vi "Blockchain test.vi"() -> ()   [LabVIEW 2013]
uses:
  JSONtext.lvlib
  <vilib>/gmath/NI_Gmath.lvlib
  <vilib>/addons/JSON API/Get Polymorphic/JSON GetSet.lvlib
  <vilib>/addons/JSON API/JSON Value/Set from JSON string.vi
  <vilib>/addons/JSON API/JSON Value/JSON Value.lvclass
  <vilib>/addons/JSON API/Variant JSON/Get as Variant.vi
  <vilib>/addons/JSON API/Variant JSON/Variant JSON.lvlib
panel:
  out "x = y? 2":T1
  out "Cluster 2":T2={"A 6"=34, "T 1"="L", "A"=3, "T 3"="", "T 4"="", "A 2"=1.23456, "T 5"="Test \"quote\",\nand newline.", "T 6"="sdfsdf", "A 3"=34, "Cluster 2"={"T 1"="SubCluster", "T 2"="Test \"quote\",\nand newline.", "A"=34, "T 3"="Test \"quote\",\nand newline.", "T 4"="Test \"quote\",\nand newline.", "A 2"=34, "T 5"="Test \"quote\",\nand newline.", "T 6"="Test \"quote\",\nand newline.", "A 3"=34}, "Array"=[1.23456, 1.23456, 1.23456, 1.23456, 1.23456, 1.23456, 1.23456, 1.23456, 1.23456, 1.23456, 1.23456, 1.23456, 2.23456]}
  in  "Other JSON Library":bool
  out "mean":dbl format="%.3p"
  out "length":i32
  out "Variant out":variant
  out "To Variant":dbl[](array[numeric]) format="%#_3p"
  in  "Cluster":T2={"A 6"=34, "T 1"="Line 1", "A"=34, "T 3"="{\"T\":123}", "T 4"="sdfsdfdsfsdf", "A 2"=1.23456, "T 5"="Test \"quote\",\nand newline.", "T 6"="sdfsdf", "A 3"=34, "Cluster 2"={"T 1"="SubCluster", "T 2"="Test \"quote\",\nand newline.", "A"=34, "T 3"="Test \"quote\",\nand newline.", "T 4"="Test \"quote\",\nand newline.", "A 2"=34, "T 5"="Test \"quote\",\nand newline.", "T 6"="Test \"quote\",\nand newline.", "A 3"=34}, "Array"=[1.23, 1.23, 1.23, 1.23, 1.23, 1.23, 1.23, 1.23, 1.23, 1.23, 2.23]}
  out "<JSON>":string
  out "error out":errorcluster
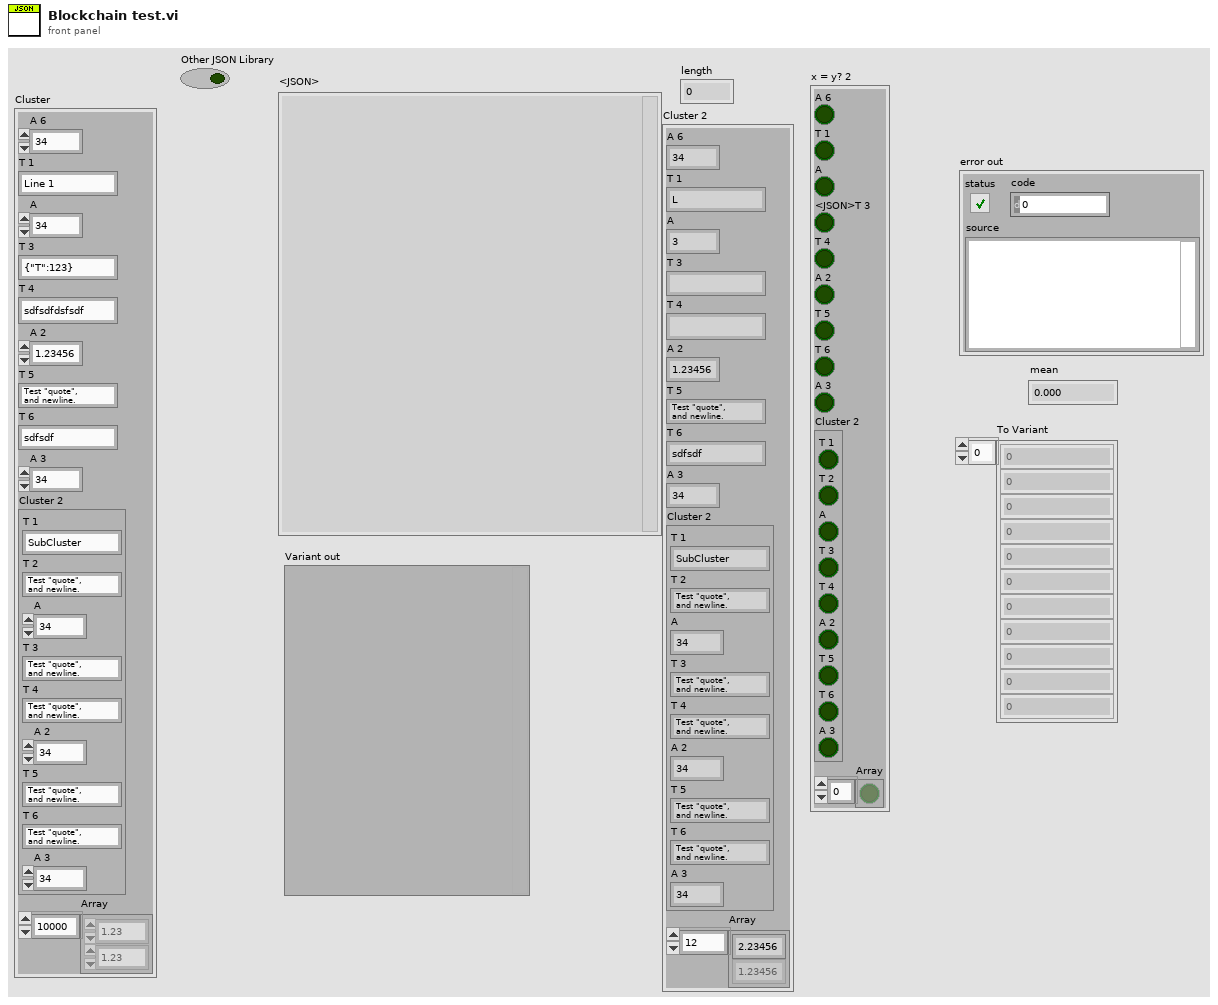
[diagram p1: front panel]
types:
  T1 = cluster{"A 6":bool, "T 1":bool, "A":bool, "<JSON>T 3":bool, "T 4":bool, "A 2":bool, "T 5":bool, "T 6":bool, "A 3":bool, "Cluster 2":cluster{"T 1":bool, "T 2":bool, "A":bool, "T 3":bool, "T 4":bool, "A 2":bool, "T 5":bool, "T 6":bool, "A 3":bool}, "Array":bool[]}
  T2 = cluster{"A 6":i32, "T 1":string, "A":i32, "T 3":string, "T 4":string, "A 2":dbl, "T 5":string, "T 6":string, "A 3":i32, "Cluster 2":cluster{"T 1":string, "T 2":string, "A":i32, "T 3":string, "T 4":string, "A 2":i32, "T 5":string, "T 6":string, "A 3":i32}, "Array":dbl[]}
  T3 = enum16{"arithmetic", "geometric", "harmonic", "trimmed", "median"}
  T4 = cluster{"A 6":bool, "T 1":bool, "A":bool, "T 3":bool, "T 4":bool, "A 2":bool, "T 5":bool, "T 6":bool, "A 3":bool, "Cluster 2":cluster{"T 1":bool, "T 2":bool, "A":bool, "T 3":bool, "T 4":bool, "A 2":bool, "T 5":bool, "T 6":bool, "A 3":bool}, "Array":bool[]}
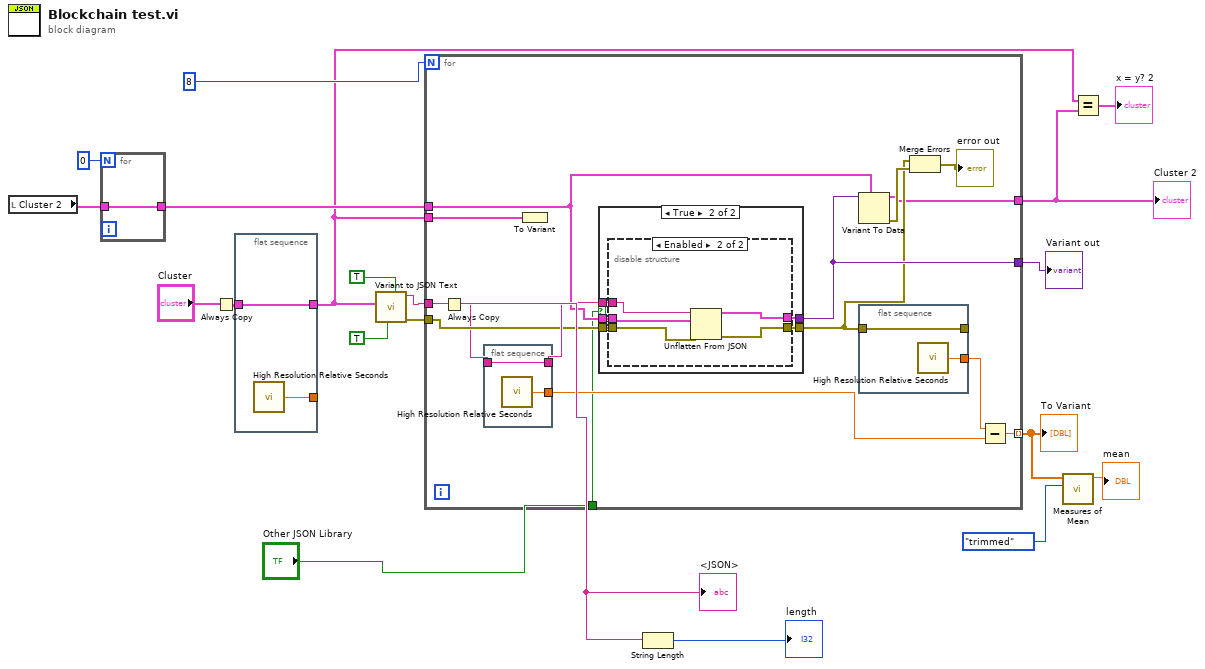
[diagram p0: block diagram]
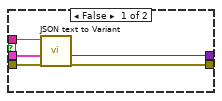
[diagram p2: hidden frame]
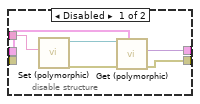
[diagram p3: hidden frame]
diagram:
  n1 = local read "Cluster 2"() -> (w16:T2)
  n2 = for {
    N: 0 -> [_]
    tunnel: [w20] -> w17
    tunnel: w16 -> [w20]
  }
  n3 = Always Copy(1:"Cluster") -> (0:w10:T2)
  n4 = flat-sequence {
    tunnel: w10 -> [w21]
    tunnel: [w22] -> _
    tunnel: [w21] -> w3
    frame #0 {
      n5 = call <vilib>:"High Resolution Relative Seconds.vi"() -> ("relative seconds"=w22:dbl)
    }
  }
  n6 = call "Variant to JSON Text.vi"("enable LabVIEW extensions? (T)"=TRUE, "Pretty Print?"=TRUE, "Variant"=w3) -> ("error out"=w11:errorcluster, "<JSON>"=w8:string)  [unwired: 7 in]
  "<JSON>" <- w8
  n7 = for {
    N: 8 -> [_]
    tunnel: [w37] -> w6 mode=indexing
    tunnel: w17 -> [w36]
    tunnel: w8 -> [w28]
    tunnel: [w23] -> w2
    tunnel: [w35] -> w14
    tunnel: w3 -> [w32]
    tunnel: w11 -> [w26]
    tunnel: "Other JSON Library" -> [w24]
    n8 = Always Copy(1:w28) -> (0:w25:string)
    n9 = flat-sequence {
      tunnel: [w60] -> w27
      tunnel: w25 -> [w60]
      tunnel: [w59] -> w31
      frame #0 {
        n10 = call <vilib>:"High Resolution Relative Seconds.vi"() -> ("relative seconds"=w59:dbl)
      }
    }
    n11 = To Variant(anything=w32) -> ()  [unwired: 1 out]
    n12 = case shown="True" w24 {
      tunnel: w36 -> [w42 w46]
      tunnel: [w41 w45] -> w35
      tunnel: [w40 w44] -> w29
      tunnel: w27 -> [w39 w47]
      tunnel: w26 -> [w38 w43]
      frame False {
        n13 = call "JSON text to Variant.vi"("error in (no error)"=w38, "Variant (Data Type)"=w42, "JSON"=w39) -> ("error out"=w40:errorcluster, "Variant out"=w41:variant)  [unwired: 7 in]
      }
      frame True {
        n14 = disable-structure shown="Enabled" {
          disable-tunnel: w47 -> [w53 w55]
          disable-tunnel: w46 -> [w52 w54]
          disable-tunnel: [w50 w58] -> w45
          disable-tunnel: [w49 w57] -> w44
          disable-tunnel: w43 -> [_ w56]
          frame Disabled {
            n15 = call-poly <vilib>:"Set (polymorphic).vi"("JSON stream"=w53) -> ("error out"=w48:errorcluster, "JSON Value out"=w51:refnum<class "JSON Value.lvclass">)  [unwired: 8 in, 1 out]
            n16 = call-poly <vilib>:"Get (polymorphic).vi"("Variant (Data Type)"=w52, "error in (no error)"=w48, "JSON in"=w51) -> ("error out"=w49:errorcluster, "Variant out"=w50:variant)  [unwired: 6 in, 1 out]
          }
          frame Enabled {
            n17 = Unflatten From JSON(JSON string=w55, type and defaults=w54, error in (no error)=w56) -> (value=w58:T2, error out=w57:errorcluster)  [unwired: 4 in]
          }
        }
      }
    }
    n18 = Variant To Data(type=w36, Variant=w35) -> (data=w23:T2, error out=w34:errorcluster)  [unwired: 1 in]
    n19 = flat-sequence {
      tunnel: [w62] -> _
      tunnel: w29 -> [w62]
      tunnel: [w61] -> w33
      frame #0 {
        n20 = call <vilib>:"High Resolution Relative Seconds.vi"() -> ("relative seconds"=w61:dbl)
      }
    }
    n21 = Merge Errors(w29, w34) -> (→"error out":errorcluster)
    n22 = Subtract(x=w33, y=w31) -> (x-y=w37:dbl)
  }
  "To Variant" <- w6
  "Variant out" <- w14
  "Cluster 2" <- w2
  n23 = String Length(string=w8) -> (length=→"length":i32)
  n24 = call <vilib>:"Measures of Mean.vi"("type"=T3."trimmed", "x array"=w6) -> ("mean value"=→"mean":dbl)  [unwired: 8 in, 1 out]
  n25 = Equal?(x=w3, y=w2) -> (x = y?=→"x = y? 2":T4)
